vi "Find All Zeros of f(x) (VI).vi"(4 "data":variant, 6 "f(x)":T1, 7 "accuracy":dbl=1e-08 format="%.2e", 8 "end":dbl=1.0 format="%.2f", 9 "start":dbl format="%.2f", 10 "algorithm":u16(ring) items=["Ridders", "Newton Raphson"], 11 "step type":u16(ring) items=["fixed function", "modified function"]) -> (0 "error":i32, 1 "ticks":u32, 2 "f(Zeros)":dbl[](array[numeric]) format="%.2f", 3 "Zeros":dbl[](array[numeric]) format="%.2f")   [LabVIEW 2020, in "NI_Gmath.lvlib"]
doc: "Determines all zeros of a 1D function in a given interval. You must manually select the polymorphic instance to use."
uses:
  <vilib>/gmath/NI_Gmath.lvlib
  <vilib>/gmath/_ref_NR.llb/functionRefnum.ctl
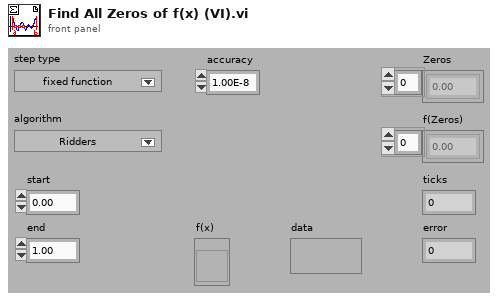
[diagram p1: front panel]
types:
  T1 = typedef "NI_Gmath.lvlib/functionRefnum.ctl" = refnum<vi>
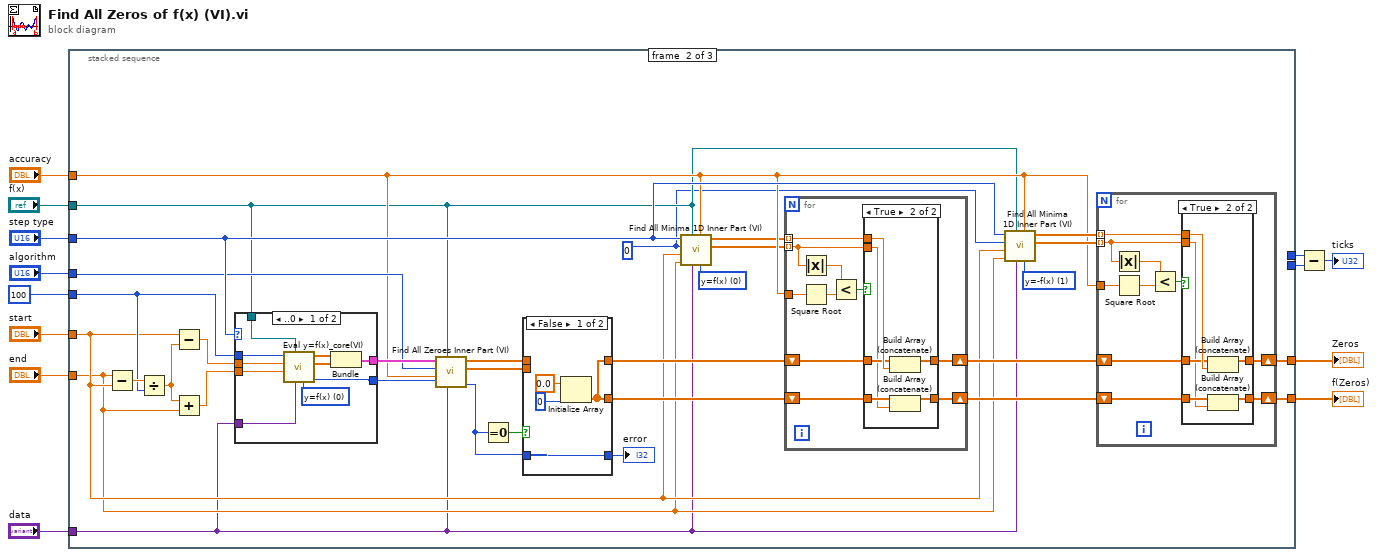
[diagram p0: block diagram]
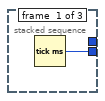
[diagram p2: hidden frame]
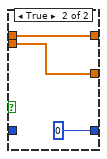
[diagram p4: hidden frame]
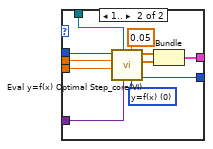
[diagram p5: hidden frame]
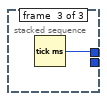
[diagram p7: hidden frame]
diagram:
  n1 = stacked-sequence {
    tunnel: u32 100 -> [_ w44 _]
    tunnel: "step type" -> [_ w26 _]
    tunnel: "data" -> [_ w22 _]
    tunnel: [_ w32 _] -> w10
    tunnel: [_ w31 _] -> w9
    tunnel: "accuracy" -> [_ w21 _]
    tunnel: "f(x)" -> [_ w20 _]
    tunnel: "start" -> [_ w24 _]
    tunnel: "end" -> [_ w23 _]
    tunnel: [w14 _ _] -> w3
    tunnel: [_ _ w111] -> w5
    tunnel: "algorithm" -> [_ w25 _]
    frame #0 {
      n2 = Tick Count (ms)() -> (millisecond timer value=w14:u32)
    }
    frame #1 {
      w15 = u16 0
      w16 = 1 items=["y=f(x)", "y=-f(x)"] ("sign")
      w17 = 0 items=["y=f(x)", "y=-f(x)"] ("sign")
      n3 = Subtract(x=w23, y=w24) -> (x-y=w46:dbl)
      n4 = Divide(x=w46, y=w44) -> (x/y=w45:dbl)
      n5 = Subtract(x=w24, y=w45) -> (x-y=w43:dbl)
      n6 = Add(x=w45, y=w23) -> (x+y=w42:dbl)
      n7 = case shown="..0" w26 {
        tunnel: w44 -> [w80 w92]
        tunnel: w43 -> [w79 w84]
        tunnel: [w81 w87] -> w41
        tunnel: w42 -> [w78 w83]
        tunnel: w22 -> [w74 w90]
        tunnel: w20 -> [w77 w91]
        tunnel: [w73 w86] -> w29
        frame ..0 {
          w72 = 0 items=["y=f(x)", "y=-f(x)"] ("sign")
          n8 = call <vilib>:"Eval y=f(x)_core(VI).vi"("sign"=w72, "data"=w74, "f(x)"=w77, "end"=w78, "start"=w79, "number of points"=w80) -> ("error out"=w73:i32, "Y Values"=w75:dbl[], "X Values"=w76:dbl[])  [unwired: 1 in, 2 out]
          n9 = Bundle("X Values"=w76, "Y Values"=w75) -> (w81:cluster{"X Values":dbl[], "Y Values":dbl[]})  [unwired: 1 out]
        }
        frame 1.. {
          w82 = 0 items=["y=f(x)", "y=-f(x)"] ("sign")
          n10 = call <vilib>:"Eval y=f(x) Optimal Step_core(VI).vi"("sign"=w82, "epsilon"=0.05, "data"=w90, "f(x)"=w91, "end"=w83, "start"=w84, "number of points"=w92) -> ("error out"=w86:i32, "Y Values"=w88:dbl[], "X Values"=w89:dbl[])  [unwired: 1 in, 1 out]
          n11 = Bundle("X Values"=w89, "Y Values"=w88) -> (w87:cluster{"X Values":dbl[], "Y Values":dbl[]})  [unwired: 1 out]
        }
      }
      n12 = call <vilib>:"Find All Zeroes Inner Part (VI).vi"("data"=w22, "f(x)"=w20, "error in"=w29, "accuracy"=w21, "algorithm"=w25, "X and Y values"=w41) -> ("error out"=w37:i32, "f(Zeroes)"=w38:dbl[], "Zeroes"=w39:dbl[])  [unwired: 3 out]
      n13 = Equal To 0?(x=w37) -> (x = 0?=w40:bool)
      n14 = case shown="False" w40 {
        tunnel: w39 -> [_ w71]
        tunnel: [w65 w71] -> w36
        tunnel: w38 -> [_ w70]
        tunnel: [w65 w70] -> w35
        tunnel: [w68 0] -> w30
        tunnel: w37 -> [w68 _]
        frame False {
          n15 = Initialize Array(0.0, 0) -> (w65:dbl[])
        }
        frame True {
        }
      }
      "error" <- w30
      n16 = call <vilib>:"Find All Minima 1D Inner Part (VI).vi"("sign"=w17, "accuracy"=w21, "data"=w22, "f(x)"=w20, "end"=w23, "start"=w24, "algorithm"=w15, "step type"=w26) -> ("f(Minima)"=w18:dbl[], "Minima"=w19:dbl[])  [unwired: 2 out]
      n17 = for {
        shift-right: [w49] -> w34
        shift-left: w36 -> [w50]
        shift-right: [w52] -> w33
        shift-left: w35 -> [w53]
        tunnel: w18 -> [w48] mode=indexing
        tunnel: w21 -> [w54]
        tunnel: w19 -> [w51] mode=indexing
        n18 = Absolute Value(x=w48) -> (abs(x)=w56:dbl)
        n19 = Square Root(x=w54) -> (sqrt(x)=w47:dbl)
        n20 = Less?(x=w56, y=w47) -> (x < y?=w55:bool)
        n21 = case shown="True" w55 {
          tunnel: w53 -> [w58 w61]
          tunnel: [w58 w60] -> w52
          tunnel: w51 -> [_ w64]
          tunnel: w50 -> [w57 w63]
          tunnel: [w57 w62] -> w49
          tunnel: w48 -> [_ w59]
          frame False {
          }
          frame True {
            n22 = Build Array (concatenate)(w63, w64) -> (w62:dbl[])
            n23 = Build Array (concatenate)(w61, w59) -> (w60:dbl[])
          }
        }
      }
      n24 = call <vilib>:"Find All Minima 1D Inner Part (VI).vi"("sign"=w16, "accuracy"=w21, "data"=w22, "f(x)"=w20, "end"=w23, "start"=w24, "algorithm"=w15, "step type"=w26) -> ("f(Minima)"=w27:dbl[], "Minima"=w28:dbl[])  [unwired: 2 out]
      n25 = for {
        shift-right: [w95] -> w32
        shift-left: w34 -> [w96]
        shift-right: [w98] -> w31
        shift-left: w33 -> [w99]
        tunnel: w27 -> [w94] mode=indexing
        tunnel: w21 -> [w100]
        tunnel: w28 -> [w97] mode=indexing
        n26 = Absolute Value(x=w94) -> (abs(x)=w102:dbl)
        n27 = Square Root(x=w100) -> (sqrt(x)=w93:dbl)
        n28 = Less?(x=w102, y=w93) -> (x < y?=w101:bool)
        n29 = case shown="True" w101 {
          tunnel: w99 -> [w104 w107]
          tunnel: [w104 w106] -> w98
          tunnel: w97 -> [_ w110]
          tunnel: w96 -> [w103 w109]
          tunnel: [w103 w108] -> w95
          tunnel: w94 -> [_ w105]
          frame False {
          }
          frame True {
            n30 = Build Array (concatenate)(w109, w110) -> (w108:dbl[])
            n31 = Build Array (concatenate)(w107, w105) -> (w106:dbl[])
          }
        }
      }
    }
    frame #2 {
      n32 = Tick Count (ms)() -> (millisecond timer value=w111:u32)
    }
  }
  "Zeros" <- w10
  "f(Zeros)" <- w9
  n33 = Subtract(x=w5, y=w3) -> (x-y=→"ticks":u32)
